vi "2015 v.02.vi"(8 "error in":errorcluster) -> (0 "error out":errorcluster)   [LabVIEW 2014]
doc: "Called before other user functions, this VI is expected to open initial I/O refnums, load in file data, and do all program initialization. Notice that the <B>error out</B> terminal is simply used for data flow. Wiring it to other structures or subVIs ensures that this VI runs first."
uses:
  <vilib>/Rock Robotics/WPI/DriverStation/WPI_DriverStationRobotMode2.ctl
  <vilib>/Rock Robotics/WPI/Joystick/WPI_JoystickDeviceEnum.ctl
  <vilib>/Rock Robotics/WPI/CAN/TalonSRX/WPI_CANTalonSRX_APIControlMode.ctl
  Robot Global Data.vi
  <vilib>/Rock Robotics/WPI/MotorControl/WPI_MotorControlOpenCANTalonSRX.vi
  <vilib>/Rock Robotics/WPI/RobotDrive/WPI_RobotDriveOpen2MotorWithCANTalonSRX.vi
  <vilib>/Rock Robotics/Network Tables/SD Write String Array.vi
  <vilib>/Rock Robotics/Network Tables/SD Write Boolean.vi
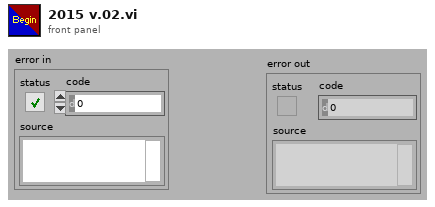
[diagram p1: front panel]
types:
  T1 = typedef "WPI_CANTalonSRX_APIControlMode.ctl" = enum8{"Percent VBus", "Speed", "Position", "Slave", "Unchanged / Invalid"}
  T2 = typedef "WPI_JoystickDeviceEnum.ctl" = enum16{"USB 0", "USB 1", "USB 2", "USB 3", "USB 4", "USB 5"}
  T3 = typedef "WPI_DriverStationRobotMode2.ctl" = enum16{"Autonomous Disabled", "Autonomous Enabled", "Teleop Disabled", "Teleop Enabled", "Disconnected", "Finish", "Test Disabled", "Test Enabled", "Emergency Stopped"}
  T4 = typedef "WPI_MotorControlDeviceRef.ctl" = cluster{"DeviceStatus":errorcluster, "Type":T5, "PWM":cluster{"Controller":T6, "PWM Channel":T7, "DeadBand":T8}, "CAN":cluster{"Device Number":u8, "Control Mode":T9, "Semaphore":T10, "Max Vout":dbl, "TalonSRX Control Mode":T1}, "Invert":bool, "TransformRef":T11, "InvTransformRef":T11}
  T5 = typedef "WPI_MotorControlType.ctl" = enum16{"PWM", "CAN", "CANTalonSRX"}
  T6 = typedef "FPGA_TypedefDigitalModule.ctl" = enum16{"Controller 1"}
  T7 = typedef "FPGA_DIOPWMChannel.ctl" = enum8{"PWM 0", "PWM 1", "PWM 2", "PWM 3", "PWM 4", "PWM 5", "PWM 6", "PWM 7", "PWM 8", "PWM 9", "PWM MXP 0", "PWM MXP 1", "PWM MXP 2", "PWM MXP 3", "PWM MXP 4", "PWM MXP 5", "PWM MXP 6", "PWM MXP 7", "PWM MXP 8", "PWM MXP 9", "Invalid"}
  T8 = typedef "WPI_PWMDeadband.ctl" = cluster{"Name":string, "maxPositivePwm":i32, "minPositivePwm":i32, "centerPwm":i32, "maxNegativePwm":i32, "minNegativePwm":i32, "angularRange":u16}
  T9 = typedef "WPI_CANJaguar_ControlMode.ctl" = enum8{"Percent VBus", "Current", "Speed", "Position", "Voltage"}
  T10 = typedef "Semaphore RefNum" = refnum<k1>
  T11 = typedef "WPI_PWMTransform_ConPane.ctl" = refnum<vi>
  T12 = typedef "WPI_RobotDriveDevRef.ctl" = cluster{"DevStatus":errorcluster, "Motors[]":T4[], "Square Inputs":bool, "Max Output":dbl}
  T13 = typedef "WPI_JoystickDevRef.ctl" = cluster{"Device":T2}
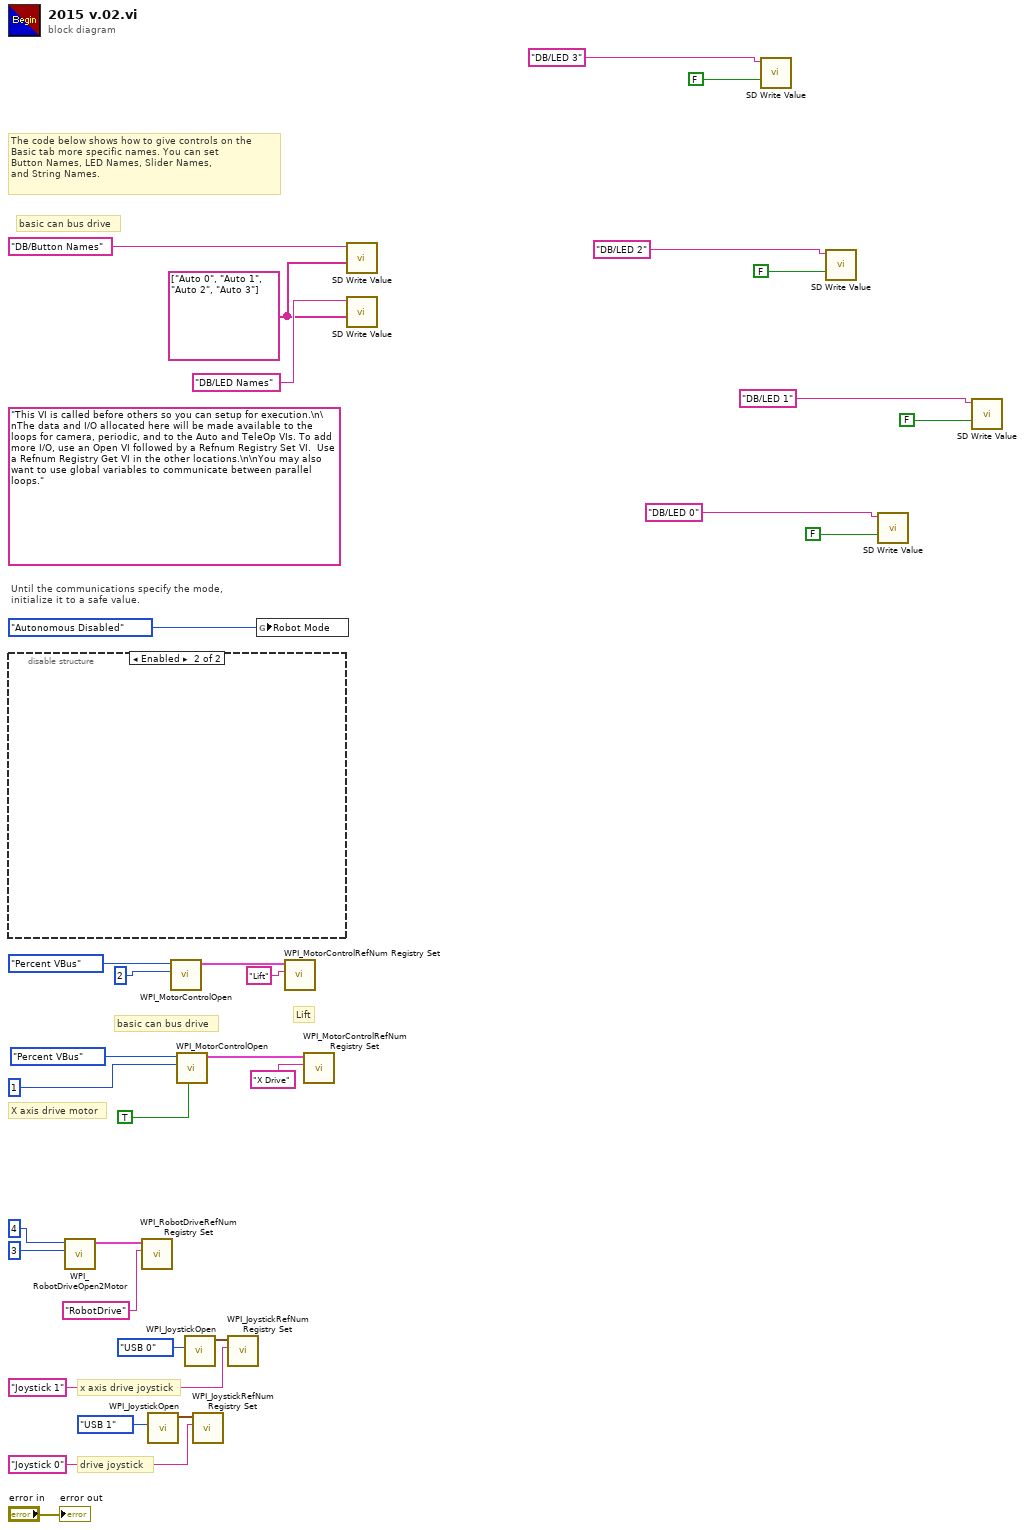
[diagram p0: block diagram]
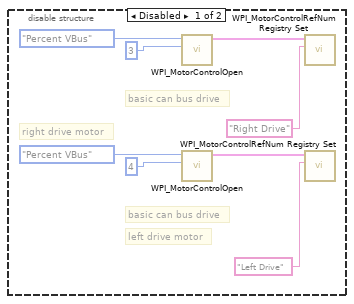
[diagram p2: hidden frame]
diagram:
  w9 = string[] ["Auto 0", "Auto 1", "Auto 2", "Auto 3"]
  (unwired) "This VI is called before others so you can setup for execution.\n\nThe data and I/O allocated here will be made available to the loops for camera, periodic, and to the Auto and TeleOp VIs. To add more I/O, use an Open VI followed by a Refnum Registry Set VI.  Use a Refnum Registry Get VI in the other locations.\n\nYou may also want to use global variables to communicate between parallel loops."
  # "X axis drive motor"
  # "basic can bus drive"
  # "Lift"
  # "basic can bus drive"
  # "x axis drive joystick"
  # "drive joystick"
  # "The code below shows how to give controls on the\nBasic tab more specific names. You can set\nButton Names, LED Names, Slider Names,\nand String Names."
  # "Until the communications specify the mode,\ninitialize it to a safe value."
  n1 = disable-structure shown="Enabled" {
    frame Disabled {
      # "left drive motor"
      # "basic can bus drive"
      # "right drive motor"
      # "basic can bus drive"
      n2 = call-poly <vilib>:"WPI_MotorControlOpen.vi"("Device Number"=u8 3, "Control Mode"=WPI_CANTalonSRX_APIControlMode."Percent VBus") -> ("MotorControlDeviceRef"=w40:T4)  [unwired: 8 in, 1 out]
      n3 = call-poly <vilib>:"WPI_MotorControlOpen.vi"("Device Number"=u8 4, "Control Mode"=WPI_CANTalonSRX_APIControlMode."Percent VBus") -> ("MotorControlDeviceRef"=w36:T4)  [unwired: 8 in, 1 out]
      n4 = call <vilib>:"WPI_MotorControlRefNum Registry Set.vi"("refnum name"="Right Drive", "MotorControlDevRef"=w40) -> ()  [unwired: 8 in, 2 out]
      n5 = call <vilib>:"WPI_MotorControlRefNum Registry Set.vi"("refnum name"="Left Drive", "MotorControlDevRef"=w36) -> ()  [unwired: 8 in, 2 out]
    }
    frame Enabled {
    }
  }
  n6 = call-poly <vilib>:"WPI_RobotDriveOpen2Motor.vi"("Right Motor"=u8 3, "Left Motor"=u8 4) -> ("RobotDriveDevRef"=w15:T12)  [unwired: 8 in, 1 out]
  n7 = call <vilib>:"WPI_RobotDriveRefNum Registry Set.vi"("refnum name"="RobotDrive", "RobotDriveDevRef"=w15) -> ()  [unwired: 8 in, 2 out]
  n8 = call <vilib>:"WPI_JoystickOpen.vi"("JoystickDevice"=WPI_JoystickDeviceEnum."USB 1") -> ("JoystickDevRef"=w30:T13)  [unwired: 10 in]
  n9 = call-poly <vilib>:"WPI_MotorControlOpen.vi"("Device Number"=u8 2, "Control Mode"=WPI_CANTalonSRX_APIControlMode."Percent VBus") -> ("MotorControlDeviceRef"=w23:T4)  [unwired: 8 in, 1 out]
  n10 = call-poly <vilib>:"WPI_MotorControlOpen.vi"("Invert"=TRUE, "Device Number"=u8 1, "Control Mode"=WPI_CANTalonSRX_APIControlMode."Percent VBus") -> ("MotorControlDeviceRef"=w20:T4)  [unwired: 7 in, 1 out]
  n11 = call <vilib>:"WPI_JoystickOpen.vi"("JoystickDevice"=WPI_JoystickDeviceEnum."USB 0") -> ("JoystickDevRef"=w25:T13)  [unwired: 10 in]
  n12 = call <vilib>:"WPI_JoystickRefNum Registry Set.vi"("refnum name"="Joystick 0", "JoystickDevRef"=w30) -> ()  [unwired: 8 in, 2 out]
  n13 = call <vilib>:"WPI_JoystickRefNum Registry Set.vi"("refnum name"="Joystick 1", "JoystickDevRef"=w25) -> ()  [unwired: 8 in, 2 out]
  n14 = global write "Robot Global Data.vi" "Robot Mode"(WPI_DriverStationRobotMode2."Autonomous Disabled" ("Robot Mode")) -> ()
  n15 = call <vilib>:"WPI_MotorControlRefNum Registry Set.vi"("refnum name"="Lift", "MotorControlDevRef"=w23) -> ()  [unwired: 8 in, 2 out]
  n16 = call <vilib>:"WPI_MotorControlRefNum Registry Set.vi"("refnum name"="X Drive", "MotorControlDevRef"=w20) -> ()  [unwired: 8 in, 2 out]
  n17 = call-poly <vilib>:"SD Write Value.vi"("String Array"=w9, "Name"="DB/Button Names") -> ()  [unwired: 8 in, 2 out]
  n18 = call-poly <vilib>:"SD Write Value.vi"("String Array"=w9, "Name"="DB/LED Names") -> ()  [unwired: 8 in, 2 out]
  n19 = call-poly <vilib>:"SD Write Value.vi"("Boolean"=FALSE, "Name"="DB/LED 3" ("refnum name")) -> ()  [unwired: 8 in, 2 out]
  n20 = call-poly <vilib>:"SD Write Value.vi"("Boolean"=FALSE, "Name"="DB/LED 2" ("refnum name")) -> ()  [unwired: 8 in, 2 out]
  n21 = call-poly <vilib>:"SD Write Value.vi"("Boolean"=FALSE, "Name"="DB/LED 0" ("refnum name")) -> ()  [unwired: 8 in, 2 out]
  n22 = call-poly <vilib>:"SD Write Value.vi"("Boolean"=FALSE, "Name"="DB/LED 1" ("refnum name")) -> ()  [unwired: 8 in, 2 out]
  "error out" <- "error in"
